vi "test Create Configuration File.vi"(8 "error in (no error)":errorcluster, 11 "TestCase in":refnum<class "Configuration Tests.lvclass">) -> (0 "error out":errorcluster, 3 "TestCase out":refnum<class "Configuration Tests.lvclass">)   [LabVIEW 2017, in "Configuration Tests.lvclass"]
uses:
  Configuration Tests.lvclass
  Configuration/Public/Controls/DSF Version Info.ctl
  Configuration/Public/Controls/DSF Plugin Info.ctl
  Configuration/Public/Controls/DSF Timing Info.ctl
  Configuration/Public/Write Item/Write Plugin.vi
  <vilib>/addons/_JKI Toolkits/VI Tester/TestCase.llb/TestCase.lvclass
  Configuration/Configuration Session.lvclass
  DSF Core.lvlib
  C:/Program Files (x86)/National Instruments/LabVIEW 2017/vi.lib/addons/_JKI Toolkits/VI Tester/TestCase.llb/TestCase.lvclass
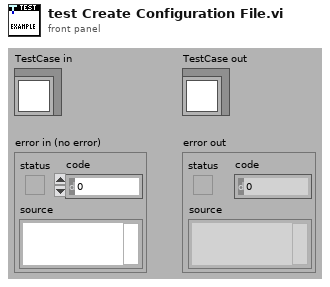
[diagram p1: front panel]
types:
  T1 = typedef "DSF Core.lvlib/DSF Plugin Info.ctl" = cluster{"type":string, "timing":T2, "group ids":string[], "settings id":string, "thread count":i32}
  T2 = typedef "DSF Core.lvlib/DSF Timing Info.ctl" = cluster{"priority":u64, "decimation":u64, "offset":u64}
  T3 = typedef "DSF Core.lvlib/DSF Version Info.ctl" = cluster{"major":u32, "minor":u32, "fix":u32, "build":string}
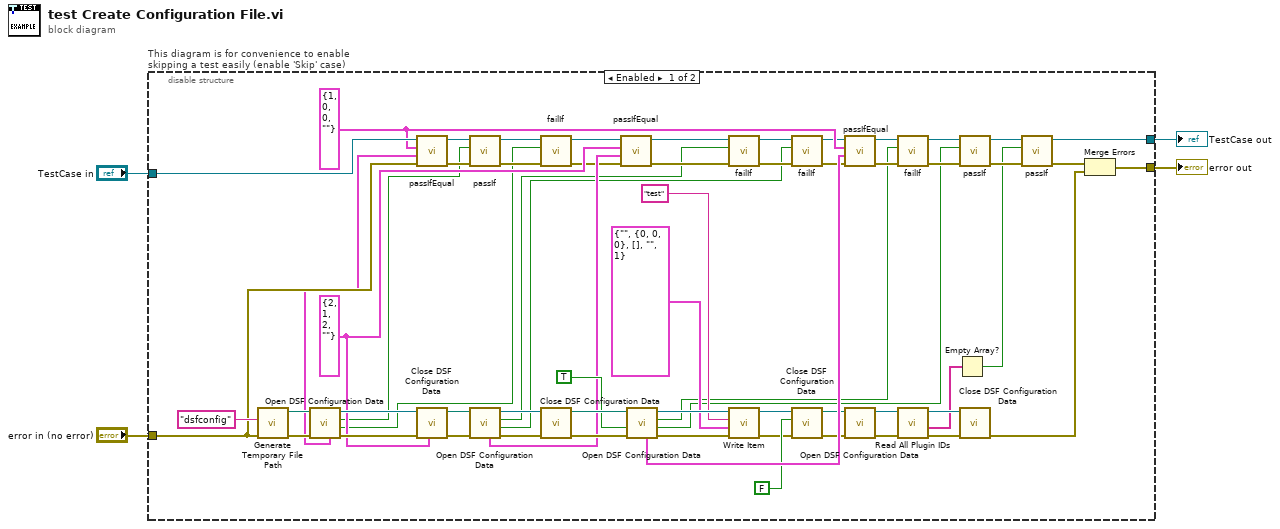
[diagram p0: block diagram]
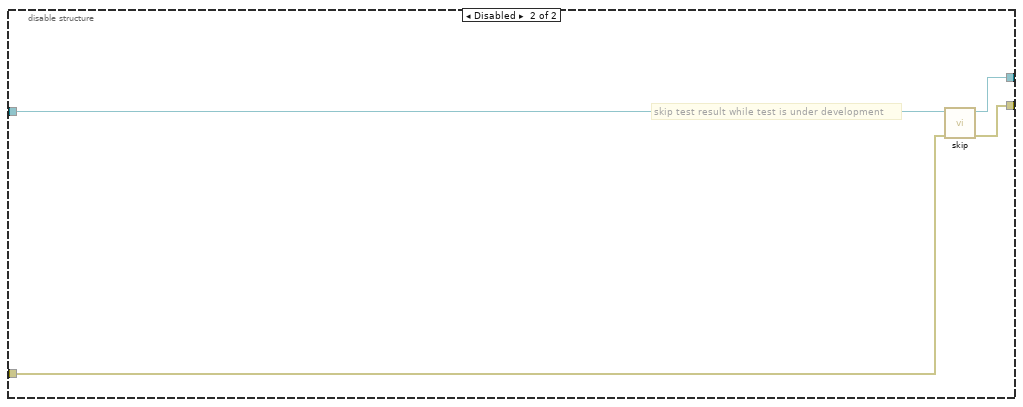
[diagram p2: hidden frame]
diagram:
  n1 = disable-structure "This diagram is for convenience to enable skipping a test easily (enable 'Skip' case)" shown="Enabled" {
    disable-tunnel: "TestCase in" -> [w63 w70]
    disable-tunnel: [w6 w68] -> w1
    disable-tunnel: [w61 w69] -> w3
    disable-tunnel: "error in (no error)" -> [w62 w67]
    frame Enabled {
      w45 = T3 {"major"=2, "minor"=1, "fix"=2, "build"=""} ("version (no change)")
      w43 = T3 {"major"=1, "minor"=0, "fix"=0, "build"=""} ("version")
      n2 = call <vilib>:"Generate Temporary File Path.vi"("error in (no error)"=w62, "Temporary File Extension (tmp)"="dsfconfig") -> ("error out"=w65:errorcluster, "Unique Temporary File Path"=w66:path)  [unwired: 8 in]
      n3 = call "Open DSF Configuration Data.vi"("error in (no error)"=w65, "dsf configuration file path"=w66) -> ("error out"=w59:errorcluster, "file replaced?"=w36:bool, "file created?"=w40:bool, "Configuration Session"=w57:refnum<class "Configuration Session.lvclass">, "version"=w44:T3)  [unwired: 5 in]
      n4 = call-dynamic "passIfEqual.vi"("error in (no error)"=w62, "y"=w44, "x"=w43, "TestCase in"=w63) -> ("error out"=w60:errorcluster, "TestCase out"=w41:refnum<class "Configuration Tests.lvclass">)  [unwired: 6 in]
      n5 = call "Close DSF Configuration Data.vi"("version (no change)"=w45, "error in (no error)"=w59, "Configuration Session"=w57) -> ("error out"=w58:errorcluster, "file path"=w56:path)  [unwired: 7 in]
      n6 = call-dynamic "passIf.vi"("error in (no error)"=w60, "pass"=w40, "TestCase in"=w41) -> ("error out"=w42:errorcluster, "TestCase out"=w38:refnum<class "Configuration Tests.lvclass">)  [unwired: 7 in]
      n7 = call "Open DSF Configuration Data.vi"("error in (no error)"=w58, "dsf configuration file path"=w56) -> ("error out"=w53:errorcluster, "file replaced?"=w15:bool, "file created?"=w19:bool, "Configuration Session"=w54:refnum<class "Configuration Session.lvclass">, "version"=w46:T3)  [unwired: 5 in]
      n8 = call-dynamic "failIf.vi"("error in (no error)"=w42, "fail"=w36, "TestCase in"=w38) -> ("error out"=w39:errorcluster, "TestCase out"=w37:refnum<class "Configuration Tests.lvclass">)  [unwired: 7 in]
      n9 = call "Close DSF Configuration Data.vi"("error in (no error)"=w53, "Configuration Session"=w54) -> ("error out"=w52:errorcluster, "file path"=w51:path)  [unwired: 8 in]
      n10 = call-dynamic "passIfEqual.vi"("error in (no error)"=w39, "y"=w46, "x"=w45, "TestCase in"=w37) -> ("error out"=w55:errorcluster, "TestCase out"=w20:refnum<class "Configuration Tests.lvclass">)  [unwired: 6 in]
      n11 = call "Open DSF Configuration Data.vi"("error in (no error)"=w52, "replace if found? (F)"=TRUE, "dsf configuration file path"=w51) -> ("error out"=w48:errorcluster, "file replaced?"=w9:bool, "file created?"=w10:bool, "Configuration Session"=w33:refnum<class "Configuration Session.lvclass">, "version"=w47:T3)  [unwired: 4 in]
      n12 = call-dynamic "failIf.vi"("error in (no error)"=w55, "fail"=w19, "TestCase in"=w20) -> ("error out"=w21:errorcluster, "TestCase out"=w17:refnum<class "Configuration Tests.lvclass">)  [unwired: 7 in]
      n13 = call-poly "Write Item.vi"("error in (no error)"=w48, "plugin values"=T1 {"type"="", "timing"={"priority"=0, "decimation"=0, "offset"=0}, "group ids"=[], "settings id"="", "thread count"=1}, "id"="test", "Configuration Session in"=w33) -> ("error out"=w34:errorcluster, "Configuration Session out"=w32:refnum<class "Configuration Session.lvclass">)  [unwired: 5 in, 1 out]
      n14 = call-dynamic "failIf.vi"("error in (no error)"=w21, "fail"=w15, "TestCase in"=w17) -> ("error out"=w18:errorcluster, "TestCase out"=w16:refnum<class "Configuration Tests.lvclass">)  [unwired: 7 in]
      n15 = call "Close DSF Configuration Data.vi"("error in (no error)"=w34, "write file if changed (T)"=FALSE, "Configuration Session"=w32) -> ("error out"=w27:errorcluster, "file path"=w29:path)  [unwired: 7 in]
      n16 = call-dynamic "passIfEqual.vi"("error in (no error)"=w18, "y"=w47, "x"=w43, "TestCase in"=w16) -> ("error out"=w49:errorcluster, "TestCase out"=w13:refnum<class "Configuration Tests.lvclass">)  [unwired: 6 in]
      n17 = call "Open DSF Configuration Data.vi"("error in (no error)"=w27, "dsf configuration file path"=w29) -> ("error out"=w28:errorcluster, "Configuration Session"=w24:refnum<class "Configuration Session.lvclass">)  [unwired: 5 in, 3 out]
      n18 = call-dynamic "failIf.vi"("error in (no error)"=w49, "fail"=w10, "TestCase in"=w13) -> ("error out"=w14:errorcluster, "TestCase out"=w11:refnum<class "Configuration Tests.lvclass">)  [unwired: 7 in]
      n19 = call "Read All Plugin IDs.vi"("error in (no error)"=w28, "Configuration Session in"=w24) -> ("error out"=w25:errorcluster, "Plugin IDs"=w22:string[], "Configuration Session out"=w23:refnum<class "Configuration Session.lvclass">)  [unwired: 7 in]
      n20 = Empty Array?(array=w22) -> (empty?=w5:bool)
      n21 = call-dynamic "passIf.vi"("error in (no error)"=w14, "pass"=w9, "TestCase in"=w11) -> ("error out"=w12:errorcluster, "TestCase out"=w7:refnum<class "Configuration Tests.lvclass">)  [unwired: 7 in]
      n22 = call "Close DSF Configuration Data.vi"("error in (no error)"=w25, "Configuration Session"=w23) -> ("error out"=w26:errorcluster)  [unwired: 8 in, 1 out]
      n23 = call-dynamic "passIf.vi"("error in (no error)"=w12, "pass"=w5, "TestCase in"=w7) -> ("error out"=w8:errorcluster, "TestCase out"=w6:refnum<class "Configuration Tests.lvclass">)  [unwired: 7 in]
      n24 = Merge Errors(w8, w26) -> (w61:errorcluster)
    }
    frame Disabled {
      # "skip test result while test is under development"
      n25 = call <vilib>:"skip.vi"("error in (no error)"=w67, "TestCase in"=w70) -> ("error out"=w69:errorcluster, "TestCase out"=w68:refnum<class "Configuration Tests.lvclass">)  [unwired: 8 in]
    }
  }
  "error out" <- w3
  "TestCase out" <- w1
